vi "P4CMD Dialog_UpdateCfgData.vi"(7 "P4Proj UIDialog FP Refs":T1, 8 "error in (no error)":errorcluster, 10 "use defaults?":bool) -> (0 "error out":errorcluster, 2 "config data out":string)   [LabVIEW 2017, in "NI_SCC_P4CMD.lvlib"]
uses:
  <vilib>/SourceControl/Providers/P4CMD/NI_SCC_P4CMD.lvlib
  <vilib>/SourceControl/Providers/P4CMD/P4CMD SCC Config Info.ctl
  <vilib>/SourceControl/support/SCCSup ConfigData Conv.ctl
  <vilib>/SourceControl/Providers/P4CMD/P4CMD Mgr Functions.ctl
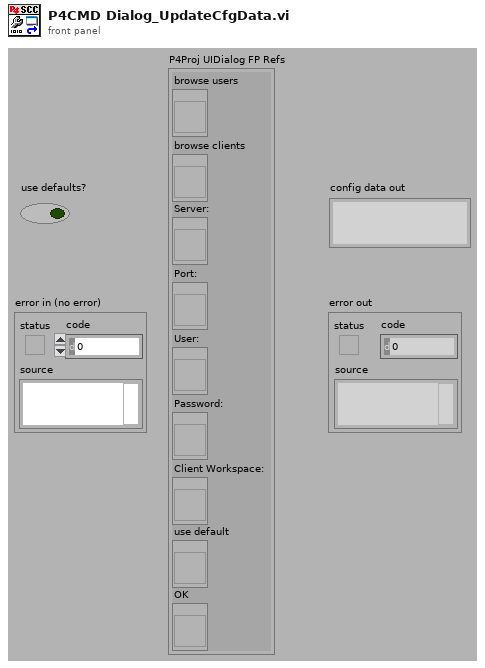
[diagram p1: front panel]
types:
  T1 = cluster{"browse users":refnum<vi>, "browse clients":refnum<vi>, "Server:":refnum<vi>, "Port:":refnum<vi>, "User:":refnum<vi>, "Password:":refnum<vi>, "Client Workspace:":refnum<vi>, "use default":refnum<vi>, "OK":refnum<vi>}
  T2 = typedef "NI_SCC_P4CMD.lvlib/P4CMD Mgr Functions.ctl" = enum16{"Init", "Open", "Set Config Opts", "Initialized?", "IsRefValid?", "Get Config Opts", "Get Global Commands", "Close", "Uninit"}
  T3 = typedef "SCCSup ConfigData Conv.ctl" = enum16{"from config data", "to config data"}
  T4 = typedef "NI_SCC_P4CMD.lvlib/P4CMD SCC Config Info.ctl" = cluster{"GBL lock on checkout?":bool, "GBL suppress dlgs?":bool, "port":string, "client":string, "user":string, "password":string}
  T5 = typedef "NI_SCC_P4CMD.lvlib/P4CMD Advanced Options.ctl" = cluster{"lock files?":bool, "suppress dialogs?":bool}
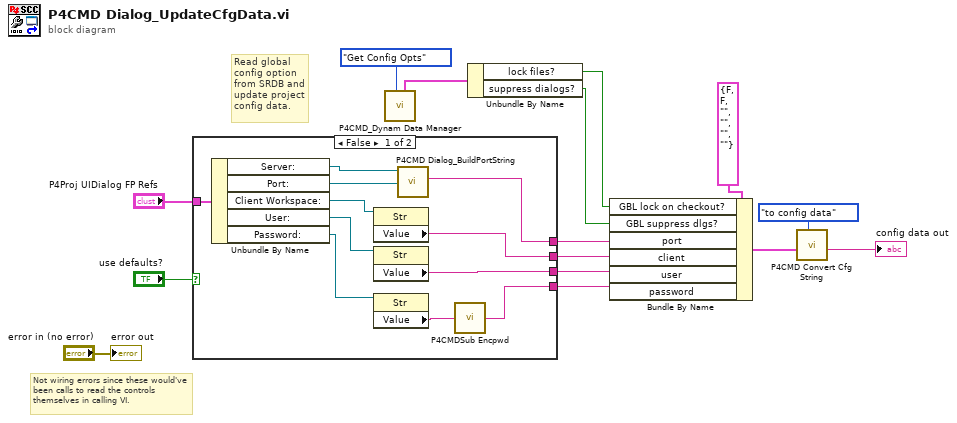
[diagram p0: block diagram]
diagram:
  # "Read global config option from SRDB and update project config data."
  # "Not wiring errors since these would've been calls to read the controls themselves in calling VI."
  n1 = case shown="False" "use defaults?" {
    tunnel: "P4Proj UIDialog FP Refs" -> [w26 _]
    tunnel: [w17 _] -> w9
    tunnel: [w21 _] -> w8
    tunnel: [w20 _] -> w7
    tunnel: [w19 _] -> w6
    frame False {
      n2 = Unbundle By Name(w26) -> ("Server:"=w18:refnum<vi>, "Port:"=w16:refnum<vi>, "Client Workspace:"=w25:refnum<vi>, "User:"=w24:refnum<vi>, "Password:"=w23:refnum<vi>)
      n3 = property class="Str"(reference=w25) -> ("Value"=w21:string)  [unwired: 1 in, 2 out]
      n4 = property class="Str"(reference=w24) -> ("Value"=w20:string)  [unwired: 1 in, 2 out]
      n5 = property class="Str"(reference=w23) -> ("Value"=w22:string)  [unwired: 1 in, 2 out]
      n6 = call <vilib>:"P4CMD Dialog_BuildPortString.vi"("Port:"=w16, "Server:"=w18) -> ("port string"=w17:string)  [unwired: 9 in]
      n7 = call <vilib>:"P4CMDSub Encpwd.vi"("input String"=w22) -> ("output String"=w19:string)  [unwired: 1 in]
    }
    frame True {
      # "If using defaults, send out empty strings since we won't use the values from the dialog."
    }
  }
  n8 = call <vilib>:"P4CMD_Dynam Data Manager.vi"("function"=P4CMD_Mgr_Functions."Get Config Opts") -> ("adv cfg options out"=w3:T5)  [unwired: 5 in, 5 out]
  n9 = Unbundle By Name(w3) -> ("lock files?"=w2:bool, "suppress dialogs?"=w1:bool)
  n10 = Bundle By Name(cluster=T4 {"GBL lock on checkout?"=FALSE, "GBL suppress dlgs?"=FALSE, "port"="", "client"="", "user"="", "password"=""} ("project details in"), "GBL lock on checkout?"=w2, "GBL suppress dlgs?"=w1, "port"=w9, "client"=w8, "user"=w7, "password"=w6) -> (w11:T4)
  n11 = call <vilib>:"P4CMD Convert Cfg String.vi"("conversion action"=SCCSup_ConfigData_Conv."to config data", "configuration details in"=w11) -> ("config data out"=→"config data out":string)  [unwired: 7 in, 2 out]
  "error out" <- "error in (no error)"
